vi "Actor Core.vi"(8 "error in":errorcluster, 11 "Datalogger Actor in":refnum<class "Datalogger Actor.lvclass">) -> (0 "error out":errorcluster, 3 "Actor out":refnum<class "Actor.lvclass">)   [LabVIEW 2018, in "Datalogger.lvlib" / "Datalogger Actor.lvclass"]
doc: "(<B>Filename</B>: Actor Framework.lvlib:Actor.lvclass:Actor Core.vi)\n\nReceives messages to the actor, reacts to them, and initiates any error handling that may shut the actor down.\n\nDescendant classes may override this VI to append parallel tasks for the actor to complete while it handles messages. Overrides use the Call Parent Method node."
uses:
  Datalogger Actor.lvclass
  C:/Program Files (x86)/National Instruments/LabVIEW 2018/vi.lib/ActorFramework/Actor/Actor.lvclass
  <vilib>/ActorFramework/Actor/Actor.lvclass
  <vilib>/ActorFramework/Actor/Actor.lvclass/Actor.ctl
  <vilib>/ActorFramework/Message Enqueuer/Message Enqueuer.lvclass/Message Enqueuer.ctl
  Datalogger Actor.lvclass/Datalogger Actor.ctl
  Datalogger Actor Messages/Log Value to File Msg/Log Value to File Msg.lvclass/Log Value to File Msg.ctl
  <vilib>/ActorFramework/Message Enqueuer/Init from Existing Queue.vi
  <vilib>/ActorFramework/Message Enqueuer/Enqueue.vi
  Datalogger Actor Messages/Log Value to File Msg/Log Value to File Msg.lvclass
  C:/Program Files (x86)/National Instruments/LabVIEW 2018/vi.lib/ActorFramework/Message/Message.lvclass
  <vilib>/ActorFramework/Stop Msg/Stop Msg.lvclass
  <vilib>/ActorFramework/Message Priority Queue/Priority Enqueue.vi
  Actor Monitor/Actor/Monitored Actor.lvclass
  <vilib>/ActorFramework/Message Enqueuer/Message Enqueuer.lvclass
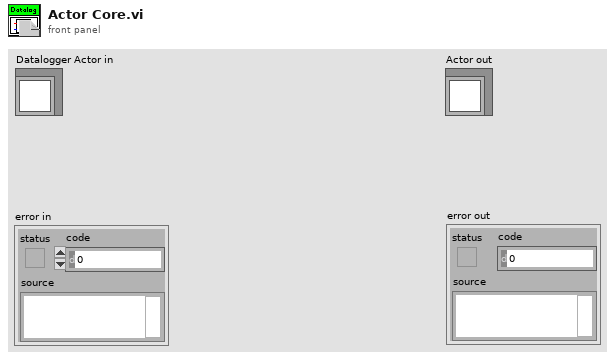
[diagram p1: front panel]
types:
  T1 = typedef "Datalogger.lvlib/Datalogger Actor.lvclass/Data Record Control.ctl" = cluster{"Timestamp":string, "Sensor Name":string, "Data (string)":string, "Units":string}
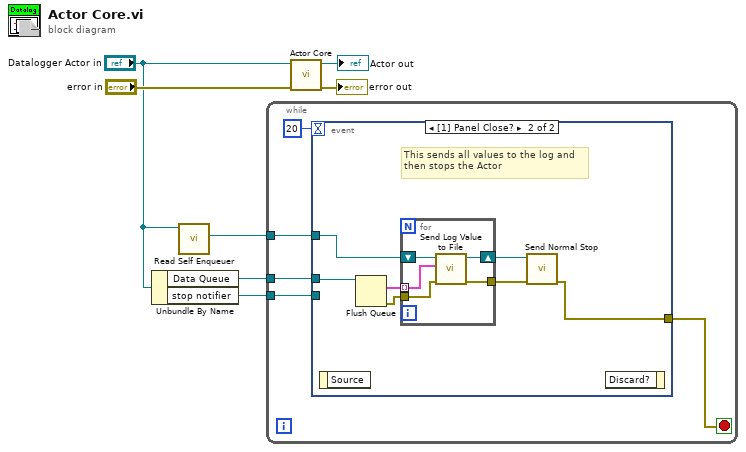
[diagram p0: block diagram]
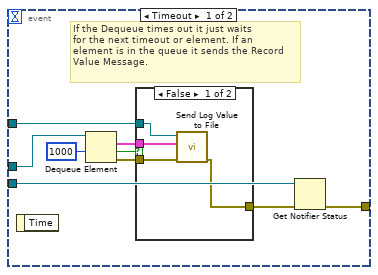
[diagram p2: hidden frame]
diagram:
  n1 = Unbundle By Name("Datalogger Actor in") -> ("Data Queue"=w1:refnum<queue>, "stop notifier"=w2:refnum<notifier>)
  n2 = call <vilib>:"Read Self Enqueuer.vi"("Actor"="Datalogger Actor in") -> ("Self Enqueuer"=w3:refnum<class "Message Enqueuer.lvclass">)  [unwired: 10 in]
  n3 = while {
    tunnel: w3 -> [w12]
    tunnel: w2 -> [w10]
    tunnel: w1 -> [w8]
    stop <- w9 stop-if-true
    n4 = event shown="[1] Panel Close?" {
      selector: _ -> [_ _]
      dyn-events: _ -> [_ _]
      timeout: 20 -> [_ _]
      tunnel: w12 -> [w19 w32]
      tunnel: w10 -> [w21 _]
      tunnel: [w20 w33] -> w9
      tunnel: w8 -> [w15 w30]
      event Timeout {
        # "If the Dequeue times out it just waits\nfor the next timeout or element. If an \nelement is in the queue it sends the Record\nValue Message."
        n5 = event-data() -> ()  [unwired: 1 in, 1 out]
        n6 = Dequeue Element(queue=w15, timeout in ms (-1)=1000) -> (element=w18:T1, timed out?=w13:bool, error out=w16:errorcluster)  [unwired: 1 in, 1 out]
        n7 = case shown="False" w13 {
          tunnel: w19 -> [w25 _]
          tunnel: w18 -> [w24 _]
          tunnel: [w23 w26] -> w17
          tunnel: w16 -> [w22 w26]
          frame False {
            n8 = call "Send Log Value to File.vi"("error in (no error)"=w22, "Data Record"=w24, "Message Enqueuer in"=w25) -> ("error out"=w23:errorcluster)  [unwired: 7 in, 1 out]
          }
          frame True {
          }
        }
        n9 = Get Notifier Status(notifier=w21, error in (no error)=w17) -> (error out=w20:errorcluster)  [unwired: 4 out]
      }
      event Panel Close? {
        # "This sends all values to the log and\nthen stops the Actor"
        n10 = event-data() -> ()  [unwired: 1 in, 1 out]
        n11 = Flush Queue(queue=w30) -> (remaining elements=w29:T1[], error out=w27:errorcluster)  [unwired: 1 in, 1 out]
        n12 = for {
          shift-right: [w37] -> w31
          shift-left: w32 -> [w38]
          tunnel: w29 -> [w36] mode=indexing
          tunnel: [w35] -> w28
          tunnel: w27 -> [w34]
          n13 = call "Send Log Value to File.vi"("error in (no error)"=w34, "Data Record"=w36, "Message Enqueuer in"=w38) -> ("error out"=w35:errorcluster, "Message Enqueuer out"=w37:refnum<class "Message Enqueuer.lvclass">)  [unwired: 7 in]
        }
        n14 = call <vilib>:"Send Normal Stop.vi"("error in (no error)"=w28, "Message Enqueuer"=w31) -> ("error out"=w33:errorcluster)  [unwired: 9 in]
        n15 = event-data() -> ()  [unwired: 2 in, 1 out]
      }
    }
  }
  n16 = call-parent "Actor Core.vi"("error in"="error in", "Actor in"="Datalogger Actor in") -> ("error out"=→"error out":errorcluster, "Actor out"=→"Actor out":refnum<class "Actor.lvclass">)  [unwired: 8 in]
